vi "Rolling Subtitles.vi"() -> ()   [LabVIEW 2011]
panel:
  in  "[user-specified font]":T1={"Font Name:"="Arial", "Size"=30, "Strikeout?"=FALSE, "Italic?"=TRUE, "Underline?"=FALSE, "Outline?"=FALSE, "Shadow?"=FALSE, "Bold?"=FALSE} caption="[用户定义字体]"
  out "new picture":picture caption="滚动字幕"
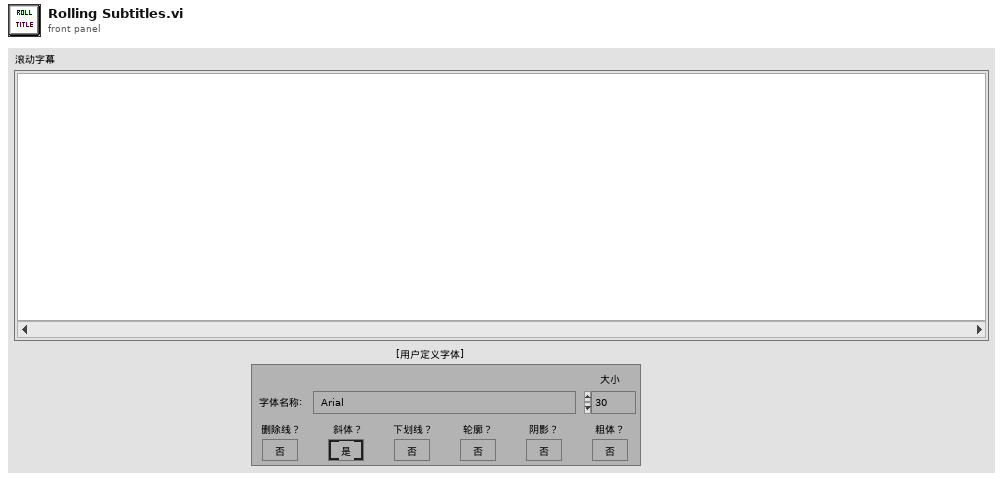
[diagram p1: front panel]
types:
  T1 = cluster{"Font Name:":string, "Size":i16, "Strikeout?":bool, "Italic?":bool, "Underline?":bool, "Outline?":bool, "Shadow?":bool, "Bold?":bool}
  T2 = enum16{"User-specified Font", "Application Font", "System Font", "Dialog Font"}
  T3 = cluster{"left":i16, "top":i16, "right":i16, "bottom":i16}
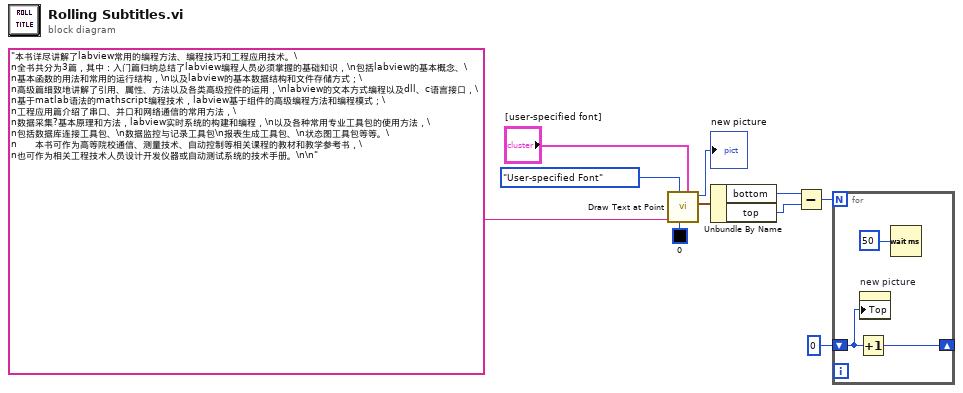
[diagram p0: block diagram]
diagram:
  n1 = call <vilib>:"Draw Text at Point.vi"("[user-specified font]"="[user-specified font]", "text color(black)"=u32 0, "desired font(Application)"=T2."User-specified Font", "text"="本书详尽讲解了labview常用的编程方法、编程技巧和工程应用技术。\n全书共分为3篇，其中：入门篇归纳总结了labview编程人员必须掌握的基础知识，\n包括labview的基本概念、\n基本函数的用法和常用的运行结构，\n以及labview的基本数据结构和文件存储方式；\n高级篇细致地讲解了引用、属性、方法以及各类高级控件的运用，\nlabview的文本方式编程以及dll、c语言接口，\n基于matlab语法的mathscript编程技术，labview基于组件的高级编程方法和编程模式；\n工程应用篇介绍了串口、并口和网络通信的常用方法，\n数据采集?基本原理和方法，labview实时系统的构建和编程，\n以及各种常用专业工具包的使用方法，\n包括数据库连接工具包、\n数据监控与记录工具包\n报表生成工具包、\n状态图工具包等等。\n　　本书可作为高等院校通信、测量技术、自动控制等相关课程的教材和教学参考书，\n也可作为相关工程技术人员设计开发仪器或自动测试系统的技术手册。\n\n") -> ("text rect"=w3:T3, "new picture"=→"new picture":picture)  [unwired: 6 in]
  n2 = Unbundle By Name(w3) -> ("bottom"=w2:i16, "top"=w1:i16)
  n3 = Subtract(x=w2, y=w1) -> (x-y=w4:i16)
  n4 = for {
    N: w4 -> [_]
    shift-right: [w13] -> _
    shift-left: i16 0 ("原点:置顶") -> [w12]
    n5 = Increment(x=w12) -> (x+1=w13:i16)
    n6 = property on="new picture" class="Pict"("Top"=w12) -> ()  [unwired: 2 in, 2 out]
    n7 = Wait (ms)(milliseconds to wait=u32 50 ("等待时间（毫秒）")) -> ()  [unwired: 1 out]
  }
